vi "getCalStructContents.vi"(11 "calType":enum16{"INTERNAL_CAL", "FULL_CAL"}(ring)) -> (0 "pdlCal?":bool, 1 "Range Strings":string[](array[string]), 3 "Calibration Information":T1 {"dutLength" format="%.2f"; "rangeArray" format="%.2f"; "minStartWL" format="%.2f"; "timeLength" format="%.2f"; "calStartWL" format="%.2f"}, 4 "Range Selection":i32)   [LabVIEW 2024]
uses:
  OVA32.dll
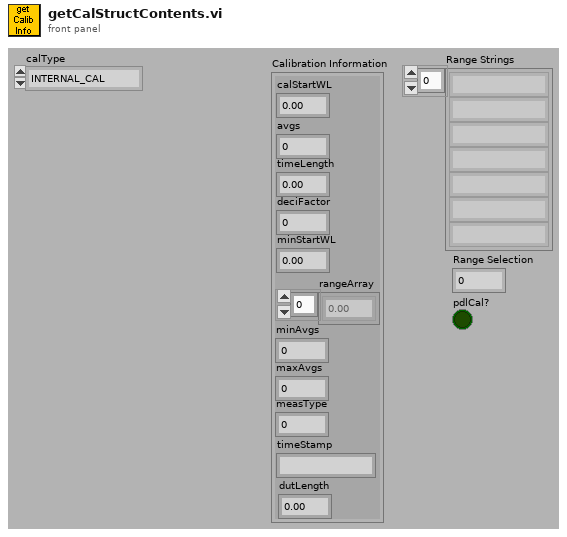
[diagram p1: front panel]
types:
  T1 = cluster{"calStartWL":dbl, "avgs":u32, "timeLength":dbl, "deciFactor":u32, "minStartWL":dbl, "rangeArray":dbl[], "minAvgs":u32, "maxAvgs":u32, "measType":u8, "timeStamp":string, "dutLength":dbl}
  T2 = cluster{"calStartWL":dbl, "avgs":u32, "timeLen":dbl, "deciFactor":u32, "minStartWL":dbl, "rangeArray":dbl[], "minAvgs":u32, "maxAvgs":u32, "measType":u8, "timeStamp":string, "dutLength":dbl}
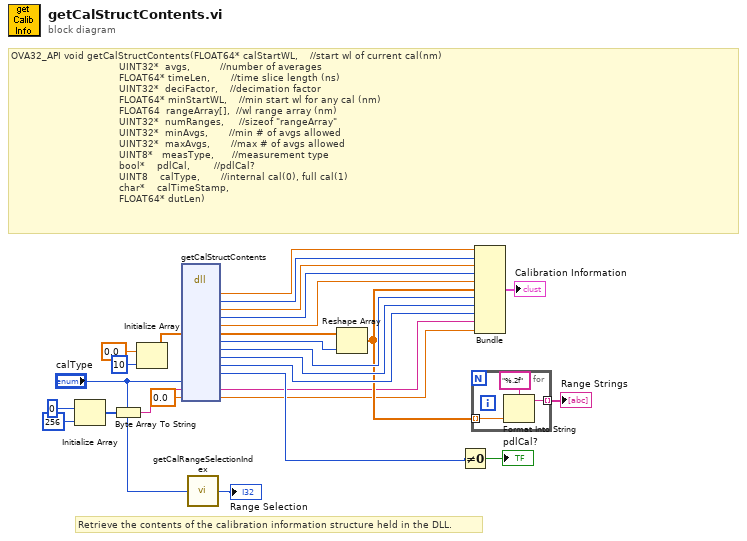
[diagram p0: block diagram]
diagram:
  # "Retrieve the contents of the calibration information structure held in the DLL."
  # "OVA32_API void getCalStructContents(FLOAT64* calStartWL,    //start wl of current cal(nm)\n                                    UINT32*  avgs,          //number of averages\n                                    FLOAT64* timeLen,       //time slice length (ns)\n                                    UINT32*  deciFactor,    //decimation factor\n                                    FLOAT64* minStartWL,    //min start wl for any cal (nm)\n                                    FLOAT64  rangeArray[],  //wl range array (nm)\n                                    UINT32*  numRanges,     //sizeof \"rangeArray\"\n                                    UINT32*  minAvgs,       //min # of avgs allowed\n                                    UINT32*  maxAvgs,       //max # of avgs allowed\n                                    UINT8*   measType,      //measurement type\n                                    bool*    pdlCal,        //pdlCal?\n                                    UINT8    calType,       //internal cal(0), full cal(1)\n                                    char*    calTimeStamp,\n                                    FLOAT64* dutLen)"
  n1 = Initialize Array(u8 0 ("Element Data"), 256 ("Dimension Size")) -> (w5:u8[])
  n2 = Byte Array To String(unsigned byte array=w5) -> (string=w2:string)
  n3 = Initialize Array(0.0 ("Element Data"), 10 ("Dimension Size")) -> (w18:dbl[])
  n4 = dll-call lib="OVA32.dll" fn="getCalStructContents"("rangeArray"=w18, "calType"="calType", "timeStamp"=w2, "dutLength"=0.0) -> ("calStartWL"=w20:dbl, "avgs"=w19:u32, "timeLen"=w23:dbl, "deciFactor"=w24:u32, "minStartWL"=w25:dbl, "rangeArray"=w13:dbl[], "numRanges"=w17:u32, "minAvgs"=w16:u32, "maxAvgs"=w15:u32, "measType"=w14:u8, "pdlCal"=w11:u8, "timeStamp"=w8:string, "dutLength"=w7:dbl)  [unwired: 15 in, 2 out]
  n5 = call "getCalRangeSelectionIndex.vi"("calType"="calType") -> ("range selection index"=→"Range Selection":u32)
  n6 = Reshape Array(w13, w17) -> (w12:dbl[])
  n7 = Not Equal To 0?(x=w11) -> (x != 0?=→"pdlCal?":bool)
  n8 = for {
    tunnel: w12 -> [w30] mode=indexing
    tunnel: [w29] -> w22 mode=indexing
    n9 = Format Into String(format string="%.2f" ("Format String"), w30) -> (resulting string=w29:string)  [unwired: 2 in, 1 out]
  }
  "Range Strings" <- w22
  n10 = Bundle("calStartWL"=w20, "avgs"=w19, "timeLen"=w23, "deciFactor"=w24, "minStartWL"=w25, "rangeArray"=w12, "minAvgs"=w16, "maxAvgs"=w15, "measType"=w14, "timeStamp"=w8, "dutLength"=w7) -> (→"Calibration Information":T2)  [unwired: 1 in]
